vi "PID for Controller Command.vi"(0 "CtrlIndex":i32, 1 "ControlArray":T1(array[cluster]), 2 "Stop CMD":dbl, 5 "CommandCluster":T3, 6 "Run?":bool, 7 "Feedback":dbl[](array[numeric]), 11 "Stability In":T2, 12 "Tolerances":dbl[](array[numeric]), 13 "Controller?":bool, 14 "Ave Feedback":dbl[](array[numeric])) -> (4 "PIdata":dbl[](array[numeric]), 8 "Output":dbl, 10 "Stable?":bool, 15 "Stability Out":T2)   [LabVIEW 2013]
uses:
  TypeDef/Command Cluster.ctl
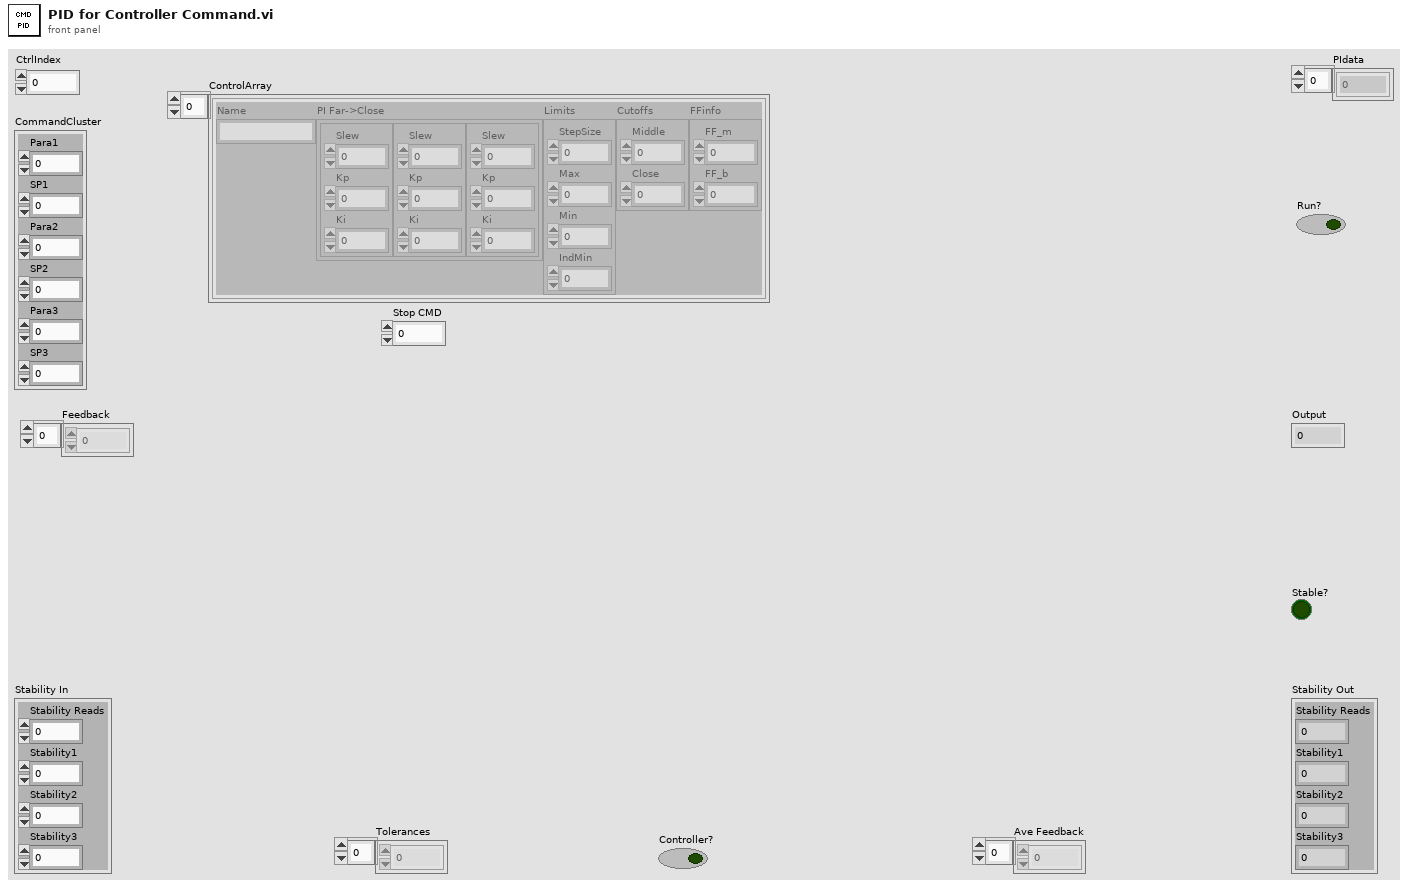
[diagram p1: front panel]
types:
  T1 = cluster{"Name":string, "PI Far->Close":cluster{"Slew":dbl, "Kp":dbl, "Ki":dbl}[], "Limits":cluster{"StepSize":dbl, "Max":dbl, "Min":dbl, "IndMin":dbl}, "Cutoffs":cluster{"Middle":dbl, "Close":dbl}, "FFinfo":cluster{"FF_m":dbl, "FF_b":dbl}}[]
  T2 = cluster{"Stability Reads":i32, "Stability1":i32, "Stability2":i32, "Stability3":i32}
  T3 = typedef "Command Cluster.ctl" = cluster{"Para1":i32, "SP1":dbl, "Para2":i32, "SP2":dbl, "Para3":i32, "SP3":dbl}
  T4 = cluster{"Name":string, "PI Far->Close":cluster{"Slew":dbl, "Kp":dbl, "Ki":dbl}[], "Limits":cluster{"StepSize":dbl, "Max":dbl, "Min":dbl, "IndMin":dbl}, "Cutoffs":cluster{"Middle":dbl, "Close":dbl}, "FFinfo":cluster{"FF_m":dbl, "FF_b":dbl}}
  T5 = cluster{"StepSize":dbl, "Max":dbl, "Min":dbl, "IndMin":dbl}
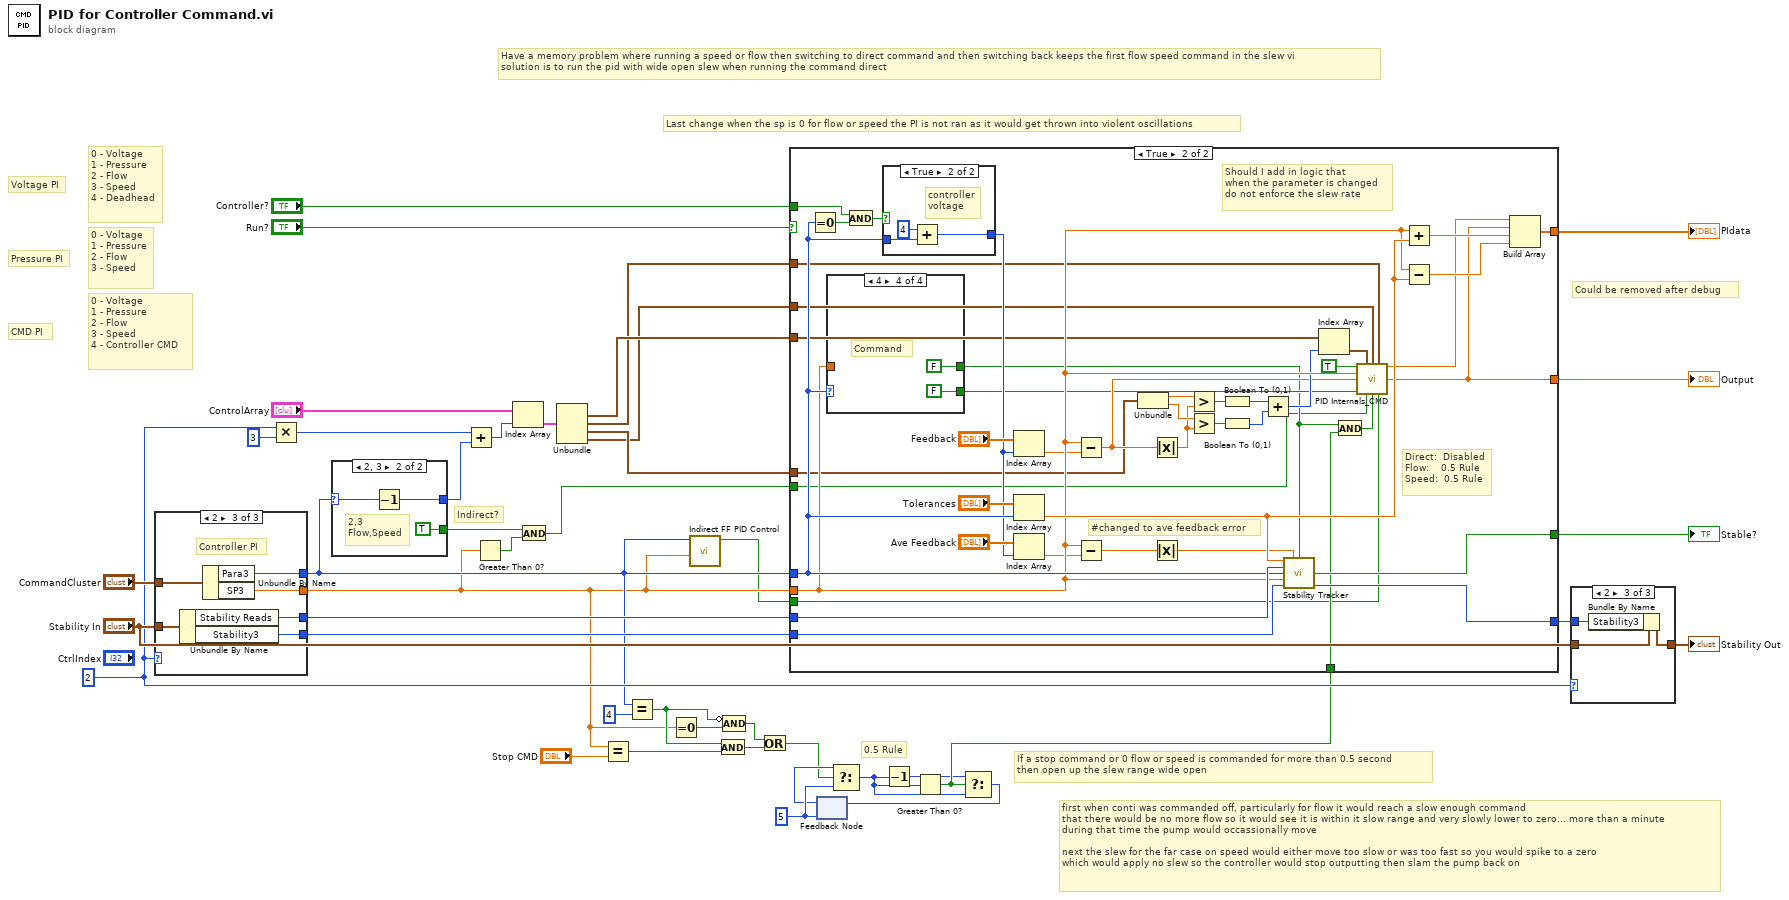
[diagram p0: block diagram]
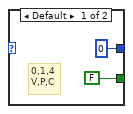
[diagram p2: hidden frame]
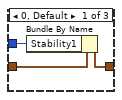
[diagram p3: hidden frame]
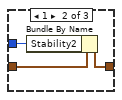
[diagram p4: hidden frame]
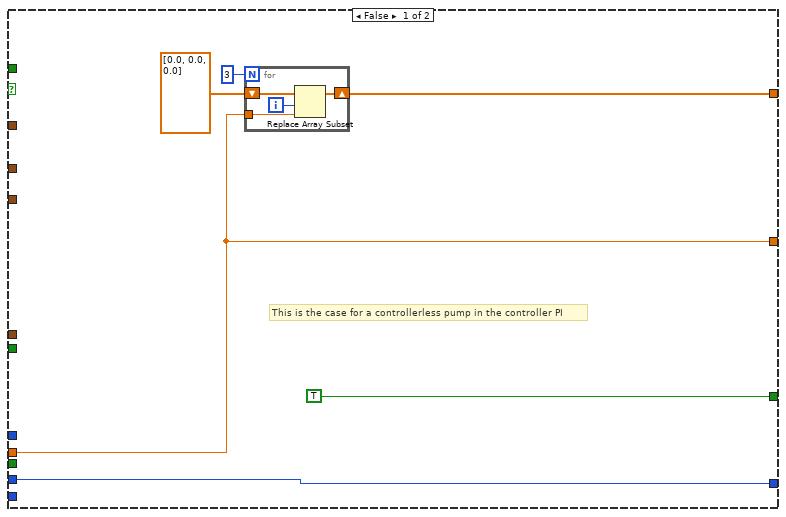
[diagram p5: hidden frame]
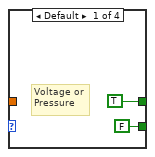
[diagram p7: hidden frame]
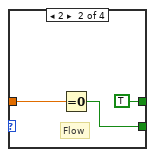
[diagram p8: hidden frame]
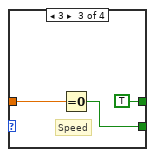
[diagram p9: hidden frame]
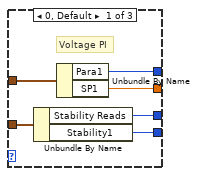
[diagram p10: hidden frame]
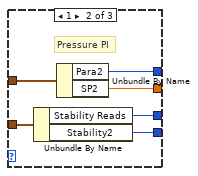
[diagram p11: hidden frame]
diagram:
  w12 = 5
  w31 = 2 ("CtrlIndex")
  # "0.5 Rule"
  # "Indirect?"
  # "Have a memory problem where running a speed or flow then switching to direct command and then switching back keeps the first flow speed command in the slew vi\nsolution is to run the pid with wide open slew when running the command direct"
  # "first when conti was commanded off, particularly for flow it would reach a slow enough command\nthat there would be no more flow so it would see it is within it slow range and very slowly lower to zero... more than a minute\nduring that time the pump would occassionally move\n\nnext the slew for the far case on speed would either move too slow or was too fast so you would spike to a zero\nwhich would apply no slew so the controller would stop outputting then slam the pump back on"
  # "If a stop command or 0 flow or speed is commanded for more than 0.5 second\nthen open up the slew range wide open"
  # "Last change when the sp is 0 for flow or speed the PI is not ran as it would get thrown into violent oscillations"
  # "Could be removed after debug"
  # "CMD PI"
  # "Pressure PI"
  # "Voltage PI"
  # "0 - Voltage\n1 - Pressure\n2 - Flow\n3 - Speed\n4 - Controller CMD"
  # "0 - Voltage\n1 - Pressure\n2 - Flow\n3 - Speed"
  # "0 - Voltage\n1 - Pressure\n2 - Flow\n3 - Speed\n4 - Deadhead"
  n1 = case shown="2" w31 {
    tunnel: "Stability In" -> [w48 w54 w60]
    tunnel: [w46 w52 w58] -> w41
    tunnel: [w47 w53 w59] -> w40
    tunnel: "CommandCluster" -> [w45 w51 w57]
    tunnel: [w44 w50 w56] -> w3
    tunnel: [w43 w49 w55] -> w2
    frame 0, Default {
      # "Voltage PI"
      n2 = Unbundle By Name(w48) -> ("Stability Reads"=w46:i32, "Stability1"=w47:i32)
      n3 = Unbundle By Name(w45) -> ("Para1"=w44:i32, "SP1"=w43:dbl)
    }
    frame 1 {
      # "Pressure PI"
      n4 = Unbundle By Name(w54) -> ("Stability Reads"=w52:i32, "Stability2"=w53:i32)
      n5 = Unbundle By Name(w51) -> ("Para2"=w50:i32, "SP2"=w49:dbl)
    }
    frame 2 {
      # "Controller PI"
      n6 = Unbundle By Name(w60) -> ("Stability Reads"=w58:i32, "Stability3"=w59:i32)
      n7 = Unbundle By Name(w57) -> ("Para3"=w56:i32, "SP3"=w55:dbl)
    }
  }
  n8 = Multiply(x=w31, y=3) -> (x*y=w29:i32)
  n9 = case shown="2, 3" w3 {
    selector: w3 -> [_ w65]
    tunnel: [0 w64] -> w21
    tunnel: [FALSE TRUE] -> w6
    frame Default {
      # "0,1,4\nV,P,C"
    }
    frame 2, 3 {
      # "2,3\nFlow,Speed"
      n10 = Decrement(x=w65) -> (x-1=w64:i32)
    }
  }
  n11 = Add(x=w29, y=w21) -> (x+y=w28:i32)
  n12 = Greater Than 0?(x=w2) -> (x > 0?=w5:bool)
  n13 = Index Array(array="ControlArray", index=w28) -> (element=w26:T4)
  n14 = And(x=w6, y=w5) -> (x .and. y?=w4:bool)
  n15 = Unbundle(w26) -> ("PI Far->Close"=w24:cluster{"Slew":dbl, "Kp":dbl, "Ki":dbl}[], "Limits"=w23:T5, "Cutoffs"=w25:cluster{"Middle":dbl, "Close":dbl}, "FFinfo"=w22:cluster{"FF_m":dbl, "FF_b":dbl})  [unwired: 1 out]
  n16 = Equal?(x=w2, y="Stop CMD") -> (x = y?=w18:bool)
  n17 = Equal?(x=w3, y=4) -> (x = y?=w17:bool)
  n18 = Equal To 0?(x=w2) -> (x = 0?=w16:bool)
  n19 = call "Indirect FF PID Control.vi"("Setpoint"=w2, "Parameter"=w3) -> ("Indirect FF"=w1:bool)  [unwired: 9 in]
  n20 = And(x=w17, y=w18) -> (x .and. y?=w14:bool)
  n21 = Compound Arithmetic op=AND(invert w17, w16) -> (w15:bool)
  n22 = Or(x=w15, y=w14) -> (x .or. y?=w10:bool)
  n23 = feedback #1(w12) -> (w11:i32)
  n24 = Select(t=w11, s=w10, f=w12) -> (s? t:f=w8:i32)
  n25 = Decrement(x=w8) -> (x-1=w7:i32)
  n26 = Greater Than 0?(x=w8) -> (x > 0?=w9:bool)
  n27 = case shown="True" "Run?" {
    tunnel: w41 -> [w70 w106]
    tunnel: w40 -> [_ w105]
    tunnel: w3 -> [_ w104]
    tunnel: w2 -> [w69 w96]
    tunnel: "Controller?" -> [_ w115]
    tunnel: [TRUE w99] -> w38
    tunnel: [w69 w85] -> w37
    tunnel: [w67 w114] -> w36
    tunnel: [w70 w107] -> w35
    tunnel: w23 -> [_ w84]
    tunnel: w25 -> [_ w89]
    tunnel: w24 -> [_ w88]
    tunnel: w22 -> [_ w87]
    tunnel: w9 -> [_ w81]
    tunnel: w4 -> [_ w77]
    tunnel: w1 -> [_ w76]
    frame False {
      # "This is the case for a controllerless pump in the controller PI"
      n28 = for {
        N: 3 -> [_]
        shift-right: [w74] -> w67
        shift-left: dbl[] [0.0, 0.0, 0.0] -> [w75]
        tunnel: w69 -> [w72]
        i -> [w73]
        n29 = Replace Array Subset(array=w75, new element=w72, index=w73) -> (w74:dbl[])
      }
    }
    frame True {
      # "Direct:  Disabled\nFlow:    0.5 Rule\nSpeed:  0.5 Rule"
      # "#changed to ave feedback error"
      # "Should I add in logic that\nwhen the parameter is changed\ndo not enforce the slew rate"
      n30 = Equal To 0?(x=w104) -> (x = 0?=w118:bool)
      n31 = case shown="4" w104 {
        tunnel: [TRUE TRUE TRUE FALSE] -> w82
        tunnel: w96 -> [_ w128 w131 _]
        tunnel: [FALSE w127 w130 FALSE] -> w90
        frame Default {
          # "Voltage or\nPressure"
        }
        frame 2 {
          # "Flow"
          n32 = Equal To 0?(x=w128) -> (x = 0?=w127:bool)
        }
        frame 3 {
          # "Speed"
          n33 = Equal To 0?(x=w131) -> (x = 0?=w130:bool)
        }
        frame 4 {
          # "Command"
        }
      }
      n34 = And(x=w115, y=w118) -> (x .and. y?=w117:bool)
      n35 = case shown="True" w117 {
        tunnel: w104 -> [w120 w123]
        tunnel: [w120 w121] -> w102
        frame False {
          # "pump\nvoltage"
        }
        frame True {
          # "controller\nvoltage"
          n36 = Add(x=4, y=w123) -> (x+y=w121:i32)
        }
      }
      n37 = Index Array(array="Feedback", index=w102) -> (element=w78:dbl)
      n38 = Index Array(array="Tolerances", index=w104) -> (element=w98:dbl)
      n39 = Index Array(array="Ave Feedback", index=w102) -> (element=w79:dbl)
      n40 = Subtract(x=w96, y=w78) -> (x-y=w91:dbl)
      n41 = Subtract(x=w96, y=w79) -> (x-y=w101:dbl)
      n42 = Unbundle(w89) -> ("Middle"=w109:dbl, "Close"=w108:dbl)
      n43 = Absolute Value(x=w91) -> (abs(x)=w100:dbl)
      n44 = Absolute Value(x=w101) -> (abs(x)=w97:dbl)
      n45 = Greater?(x=w109, y=w100) -> (0:w113:bool)
      n46 = Greater?(x=w108, y=w100) -> (0:w112:bool)
      n47 = Boolean To (0,1)(Boolean=w113) -> (0, 1=w111:i16)
      n48 = Boolean To (0,1)(Boolean=w112) -> (0, 1=w110:i16)
      n49 = Add(x=w111, y=w110) -> (x+y=w93:i16)
      n50 = call "Stability Tracker.vi"("Tolerance"=w98, "AbsError"=w97, "PI Running?"=w82, "ReqReads"=w106, "Parameter"=w104, "Setpoint"=w96, "StabilityCount In"=w105) -> ("Stable?"=w99:bool, "StabilityCount Out"=w107:i32)  [unwired: 6 in, 1 out]
      n51 = Index Array(array=w88, index=w93) -> (element=w92:cluster{"Slew":dbl, "Kp":dbl, "Ki":dbl})
      n52 = And(x=w82, y=w81) -> (x .and. y?=w80:bool)
      n53 = call "PID Internals_CMD.vi"("Run PI?"=TRUE, "PIcluster"=w92, "FFcluster"=w87, "LimitCluster"=w84, "SP"=w96, "Error"=w91, "RevCtrlZero"=w90, "IndirectMin?"=w77, "ApplySlew"=w80, "Indirect FF"=w76) -> ("PreSlew"=w86:dbl, "Output"=w85:dbl)  [unwired: 4 in]
      n54 = Add(x=w96, y=w98) -> (x+y=w95:dbl)
      n55 = Subtract(x=w96, y=w98) -> (x-y=w94:dbl)
      n56 = Build Array(w86, w85, w95, w94) -> (w114:dbl[])
    }
  }
  "Stable?" <- w38
  "Output" <- w37
  "PIdata" <- w36
  n57 = Select(t=w7, s=w9, f=w8) -> (s? t:f=w13:i32)
  n58 = feedback-in #1(w13) -> ()
  n59 = case shown="2" w31 {
    tunnel: "Stability In" -> [w135 w138 w141]
    tunnel: [w134 w137 w140] -> w39
    tunnel: w35 -> [w136 w139 w142]
    frame 0, Default {
      n60 = Bundle By Name(cluster=w135, "Stability1"=w136) -> (w134:T2)
    }
    frame 1 {
      n61 = Bundle By Name(cluster=w138, "Stability2"=w139) -> (w137:T2)
    }
    frame 2 {
      n62 = Bundle By Name(cluster=w141, "Stability3"=w142) -> (w140:T2)
    }
  }
  "Stability Out" <- w39
